vi "ConfigFileExists.vi"(11 "path":path) -> ()   [LabVIEW 2018]
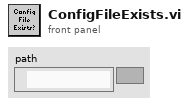
[diagram p1: front panel]
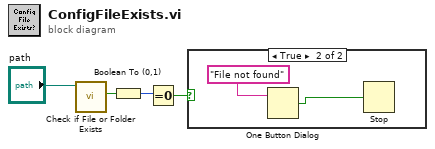
[diagram p0: block diagram]
diagram:
  n1 = call <vilib>:"Check if File or Folder Exists.vi"("path"="path") -> ("file or folder exists?"=w2:bool)  [unwired: 8 in, 2 out]
  n2 = Boolean To (0,1)(Boolean=w2) -> (0, 1=w3:i16)
  n3 = Equal To 0?(x=w3) -> (x = 0?=w4:bool)
  n4 = case shown="True" w4 {
    frame False {
    }
    frame True {
      n5 = One Button Dialog(message="File not found") -> (true=w5:bool)  [unwired: 1 in]
      n6 = Stop(stop? (T)=w5) -> ()
    }
  }
